vi "Replace Line.vi"(8 "error in (no error)":errorcluster, 9 "New Line":T1, 10 "Line Name":string, 11 "RT Resource Usage configuration in":refnum<class "RT Resource Usage configuration.lvclass">) -> (0 "error out":errorcluster, 3 "RT Resource Usage configuration out":refnum<class "RT Resource Usage configuration.lvclass">)   [LabVIEW 2017, in "RT Resource Usage configuration.lvclass"]
uses:
  RT Resource Usage configuration.lvclass
  <vilib>/NI/Tag Bus Module Framework/channel/TBM channel.lvclass
  RT Resource Usage configuration.lvclass/RT Resource Usage configuration.ctl
panel:
  out "Old Line":T1
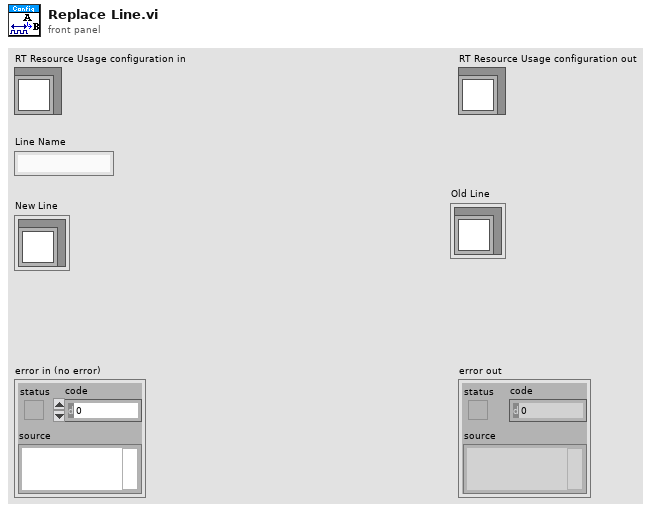
[diagram p1: front panel]
types:
  T1 = cluster{"channel":refnum<class "TBM channel.lvclass">}
  T2 = cluster{"channel":refnum<class "TBM channel.lvclass">}[]
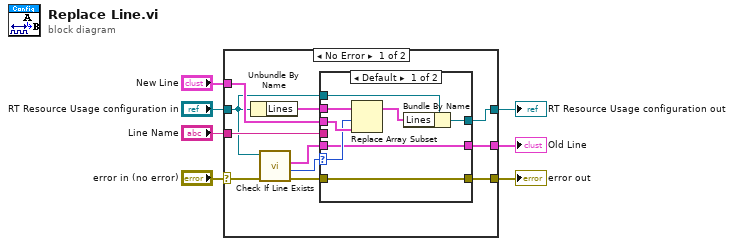
[diagram p0: block diagram]
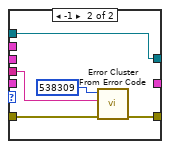
[diagram p2: hidden frame]
diagram:
  n1 = case shown="No Error" "error in (no error)" {
    selector: "error in (no error)" -> [w12 w33]
    tunnel: [w17 w33] -> w6
    tunnel: [w18 w32] -> w5
    tunnel: "RT Resource Usage configuration in" -> [w9 w32]
    tunnel: "Line Name" -> [w16 _]
    tunnel: "New Line" -> [w15 _]
    tunnel: [w13 _] -> w4
    frame No Error {
      n2 = Unbundle By Name(w9) -> ("Lines"=w14:T2)
      n3 = call-dynamic "Check If Line Exists.vi"("error in (no error)"=w12, "RT Resource Usage configuration in"=w9) -> ("error out"=w11:errorcluster, "index"=w10:i32, "Line"=w8:T1)  [unwired: 5 in, 2 out]
      n4 = case shown="Default" w10 {
        selector: w10 -> [w20 _]
        tunnel: w9 -> [w26 w31]
        tunnel: [w25 w31] -> w18
        tunnel: w14 -> [w21 _]
        tunnel: w15 -> [w23 _]
        tunnel: w16 -> [_ w29]
        tunnel: w11 -> [w22 w28]
        tunnel: [w22 w27] -> w17
        tunnel: [w19 _] -> w13
        tunnel: w8 -> [w19 _]
        frame Default {
          n5 = Replace Array Subset(array=w21, new element=w23, index=w20) -> (w24:T2)
          n6 = Bundle By Name(cluster=w26, "Lines"=w24) -> (w25:refnum<class "RT Resource Usage configuration.lvclass">)
        }
        frame -1 {
          n7 = call <vilib>:"Error Cluster From Error Code.vi"("error in (no error)"=w28, "error message (\"\")"=w29, "error code (0)"=538309) -> ("error out"=w27:errorcluster)  [unwired: 6 in]
        }
      }
    }
    frame Error {
    }
  }
  "error out" <- w6
  "RT Resource Usage configuration out" <- w5
  "Old Line" <- w4
